vi "Comments.Add Experiment Description.vi"(7 "error in (no error)":errorcluster, 10 "Control Experiment":refnum<class "Control Experiment.lvclass">) -> (0 "error out":errorcluster, 3 "Control Experiment out":refnum<class "Control Experiment.lvclass">)   [LabVIEW 2016, in "Control Experiment.lvclass"]
uses:
  Control Experiment.lvclass
  Control Experiment.lvclass/Control Experiment.ctl
panel:
  out "concatenated string":string
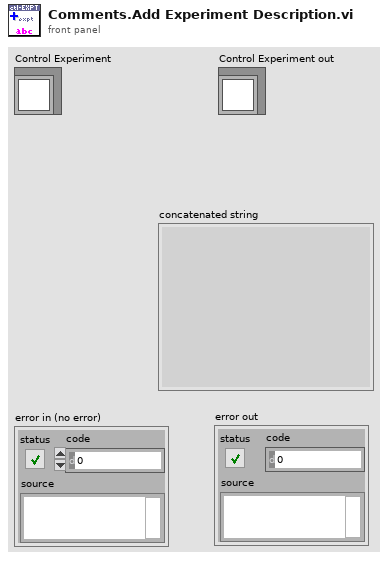
[diagram p1: front panel]
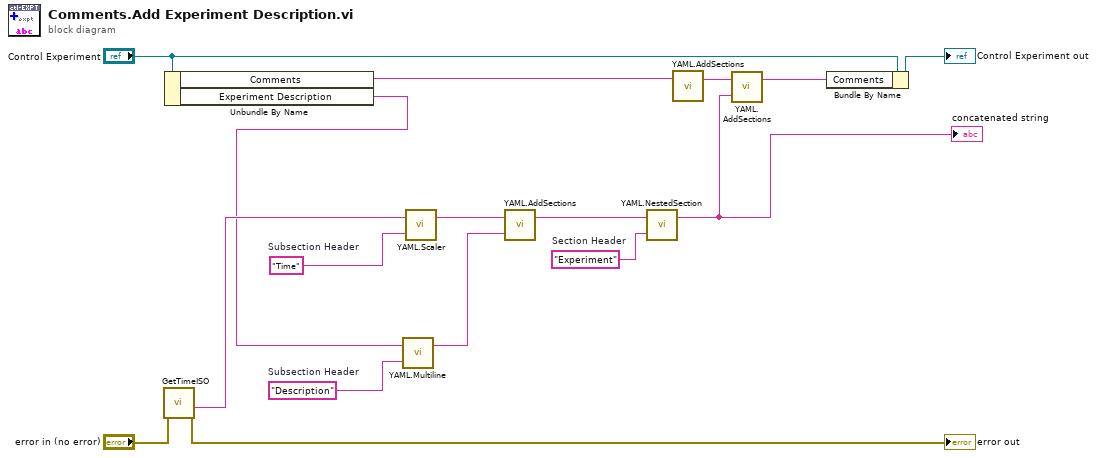
[diagram p0: block diagram]
diagram:
  w6 = "Description"  # Subsection Header
  w7 = "Time"  # Subsection Header
  w5 = "Experiment"  # Section Header
  n1 = call "GetTimeISO.vi"("error in (no error)"="error in (no error)") -> ("error out"=→"error out":errorcluster, "ISO 8601 date-time string"=w8:string)  [unwired: 8 in, 1 out]
  n2 = Unbundle By Name("Control Experiment") -> ("Comments"=w2:string, "Experiment Description"=w4:string)
  n3 = call "YAML.Multiline.vi"("Key"=w6, "Multiline"=w4) -> ("Output"=w10:string)  [unwired: 1 in]
  n4 = call "YAML.Scaler.vi"("Key"=w7, "Scaler"=w8) -> ("Output"=w12:string)  [unwired: 1 in]
  n5 = call "YAML.AddSections.vi"("Section 2"=w10, "Section 1"=w12) -> ("Output"=w9:string)  [unwired: 1 in]
  n6 = call "YAML.NestedSection.vi"("Section Key"=w5, "Nested Section"=w9) -> ("String"=w1:string)  [unwired: 1 in]
  "concatenated string" <- w1
  n7 = call "YAML.AddSections.vi"("Section 1"=w2) -> ("Output"=w3:string)  [unwired: 2 in]
  n8 = call "YAML.AddSections.vi"("Section 2"=w1, "Section 1"=w3) -> ("Output"=w11:string)  [unwired: 1 in]
  n9 = Bundle By Name(cluster="Control Experiment", "Comments"=w11) -> (→"Control Experiment out":refnum<class "Control Experiment.lvclass">)
